vi "AMLUTwaveselHD2.vi"(0 "AM Freq Hz":dbl=1000.0, 5 "Peak Power":dbl=20.0, 7 "Min Power":dbl=10.0, 9 "Wave Shape":u8(ring) items=["Sine", "Ramp", "Triangle"], 12 "Linear in?":u8(ring) items=["Linear in dB", "Linear in Volts"]) -> (4 "Waveform":dbl[](graph), 8 "Actual Freq":dbl=1000.0, 13 "LUTsize":u8=32, 15 "powerout":string)   [LabVIEW 2012]
panel:
  out "stdam":u16
  # "dBm"
  # "dBm"
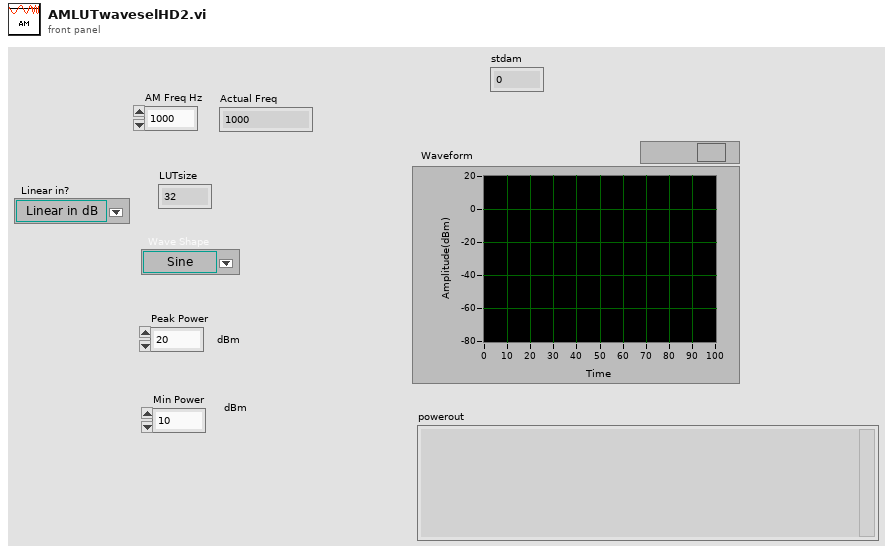
[diagram p1: front panel]
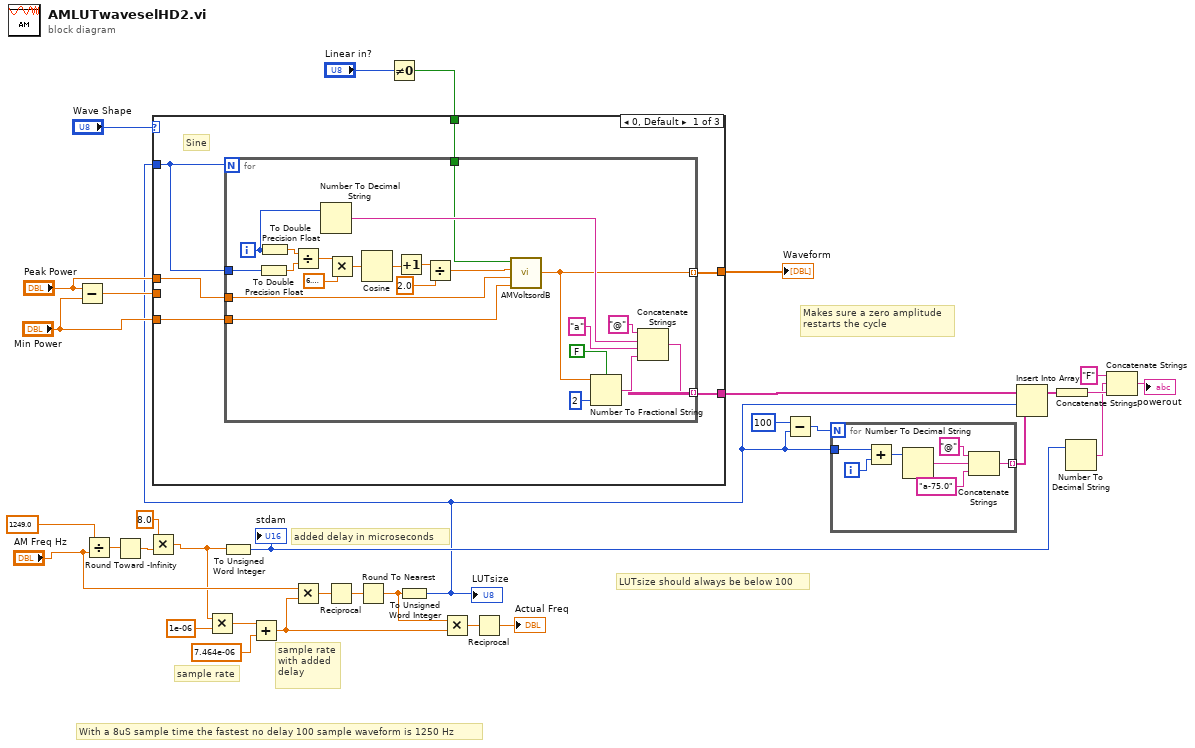
[diagram p0: block diagram]
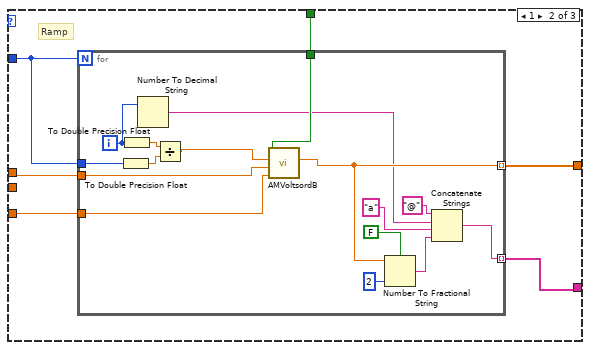
[diagram p2: hidden frame]
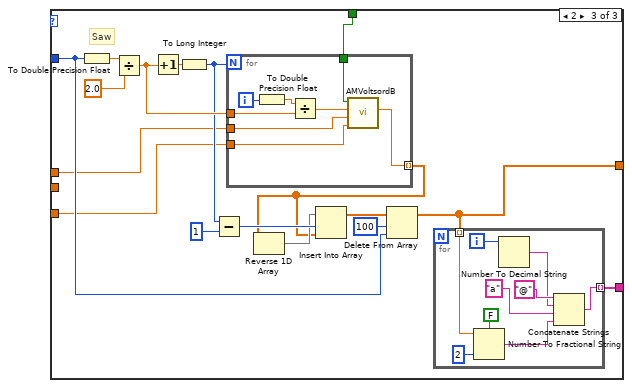
[diagram p3: hidden frame]
diagram:
  # "With a 8uS sample time the fastest no delay 100 sample waveform is 1250 Hz"
  # "LUTsize should always be below 100"
  # "added delay in microseconds"
  # "sample rate\nwith added\ndelay"
  # "sample rate"
  # "Makes sure a zero amplitude\nrestarts the cycle"
  n1 = Subtract(x="Peak Power", y="Min Power") -> (x-y=w32:dbl)
  n2 = Divide(x=1249.0, y="AM Freq Hz") -> (x/y=w11:dbl)
  n3 = Round Toward -Infinity(1:w11) -> (0:w10:dbl)
  n4 = Multiply(x=8.0, y=w10) -> (x*y=w9:dbl)
  n5 = Multiply(x=w9, y=1e-06) -> (x*y=w21:dbl)
  n6 = To Unsigned Word Integer(number=w9) -> (unsigned 16bit integer=w24:u16)
  "stdam" <- w24
  n7 = Add(x=w21, y=7.464e-06 ("x")) -> (x+y=w13:dbl)
  n8 = Multiply(x="AM Freq Hz", y=w13) -> (x*y=w19:dbl)
  n9 = Reciprocal(x=w19) -> (1/x=w18:dbl)
  n10 = Round To Nearest(number=w18) -> (nearest integer value=w14:dbl)
  n11 = Not Equal To 0?(x="Linear in?") -> (x != 0?=w5:bool)
  n12 = To Unsigned Word Integer(number=w14) -> (unsigned 16bit integer=w2:u16)
  "LUTsize" <- w2
  n13 = case shown="0, Default" "Wave Shape" {
    tunnel: [w38 w67 w89] -> w7
    tunnel: w2 -> [w39 w66 w92]
    tunnel: "Min Power" -> [w37 w65 w90]
    tunnel: [w36 w64 w88] -> w30
    tunnel: w32 -> [_ _ _]
    tunnel: w5 -> [w35 w63 w86]
    tunnel: "Peak Power" -> [w34 w62 w87]
    frame 0, Default {
      # "Sine"
      n14 = for {
        N: w39 -> [_]
        tunnel: [w42] -> w38 mode=indexing
        tunnel: w39 -> [w56]
        tunnel: w37 -> [w49]
        tunnel: [w52] -> w36 mode=indexing
        tunnel: w35 -> [w51]
        tunnel: w34 -> [w50]
        i -> [w55]
        n15 = To Double Precision Float(number=w56) -> (double precision float=w57:dbl)
        n16 = To Double Precision Float(number=w55) -> (double precision float=w58:dbl)
        n17 = Divide(x=w58, y=w57) -> (x/y=w61:dbl)
        n18 = Number To Decimal String(number=w55) -> (decimal integer string=w54:string)  [unwired: 1 in]
        n19 = Multiply(x=w61, y=6.283185307179586) -> (x*y=w59:dbl)
        n20 = Cosine(x=w59) -> (cos(x)=w48:dbl)
        n21 = Increment(x=w48) -> (x+1=w47:dbl)
        n22 = Divide(x=w47, y=2.0) -> (x/y=w45:dbl)
        n23 = call "AMVoltsordB.vi"("Min Power"=w49, "Peak Power"=w50, "Signal In"=w45, "Linear?"=w51) -> ("Out"=w42:dbl)  [unwired: 7 in]
        n24 = Number To Fractional String(use system decimal point (T)=FALSE, number=w42, precision (6)=i16 2) -> (F-format string=w43:string)  [unwired: 1 in]
        n25 = Concatenate Strings("@" ("string"), w54, "a" ("string"), w43) -> (w52:string)
      }
    }
    frame 1 {
      # "Ramp"
      n26 = for {
        N: w66 -> [_]
        tunnel: [w70] -> w67 mode=indexing
        tunnel: w66 -> [w81]
        tunnel: w62 -> [w78]
        tunnel: w65 -> [w79]
        tunnel: [w68] -> w64 mode=indexing
        tunnel: w63 -> [w77]
        i -> [w80]
        n27 = To Double Precision Float(number=w81) -> (double precision float=w82:dbl)
        n28 = To Double Precision Float(number=w80) -> (double precision float=w83:dbl)
        n29 = Number To Decimal String(number=w80) -> (decimal integer string=w69:string)  [unwired: 1 in]
        n30 = Divide(x=w83, y=w82) -> (x/y=w76:dbl)
        n31 = call "AMVoltsordB.vi"("Min Power"=w79, "Peak Power"=w78, "Signal In"=w76, "Linear?"=w77) -> ("Out"=w70:dbl)  [unwired: 7 in]
        n32 = Number To Fractional String(use system decimal point (T)=FALSE, number=w70, precision (6)=i16 2) -> (F-format string=w73:string)  [unwired: 1 in]
        n33 = Concatenate Strings("@" ("string"), w69, "a" ("string"), w73) -> (w68:string)
      }
    }
    frame 2 {
      # "Saw"
      n34 = To Double Precision Float(number=w92) -> (double precision float=w100:dbl)
      n35 = Divide(x=w100, y=2.0) -> (x/y=w97:dbl)
      n36 = Increment(x=w97) -> (x+1=w98:dbl)
      n37 = To Long Integer(number=w98) -> (32bit integer=w96:i32)
      n38 = Subtract(x=w96, y=1) -> (x-y=w95:i32)
      n39 = for {
        N: w96 -> [_]
        tunnel: [w110] -> w84 mode=indexing
        tunnel: w97 -> [w115]
        tunnel: w87 -> [w112]
        tunnel: w90 -> [w113]
        tunnel: w86 -> [w111]
        i -> [w116]
        n40 = To Double Precision Float(number=w116) -> (double precision float=w117:dbl)
        n41 = Divide(x=w117, y=w115) -> (x/y=w114:dbl)
        n42 = call "AMVoltsordB.vi"("Min Power"=w113, "Peak Power"=w112, "Signal In"=w114, "Linear?"=w111) -> ("Out"=w110:dbl)  [unwired: 7 in]
      }
      n43 = Reverse 1D Array(array=w84) -> (reversed array=w85:dbl[])
      n44 = Insert Into Array(array=w85, index=w95, new element=w84) -> (w93:dbl[])
      n45 = Delete From Array(array=w93, length=100, index=w92) -> (array with subset deleted=w89:dbl[])  [unwired: 1 out]
      n46 = for {
        tunnel: w89 -> [w102] mode=indexing
        tunnel: [w107] -> w88 mode=indexing
        i -> [w109]
        n47 = Number To Fractional String(use system decimal point (T)=FALSE, number=w102, precision (6)=i16 2) -> (F-format string=w101:string)  [unwired: 1 in]
        n48 = Number To Decimal String(number=w109) -> (decimal integer string=w106:string)  [unwired: 1 in]
        n49 = Concatenate Strings("@" ("string"), w106, "a" ("string"), w101) -> (w107:string)
      }
    }
  }
  "Waveform" <- w7
  n50 = Multiply(x=w14, y=w13) -> (x*y=w17:dbl)
  n51 = Reciprocal(x=w17) -> (1/x=→"Actual Freq":dbl)
  n52 = Subtract(x=u8 100 ("y"), y=w2) -> (x-y=w1:u16)
  n53 = for {
    N: w1 -> [_]
    tunnel: [w119] -> w4 mode=indexing
    tunnel: w2 -> [w118]
    i -> [w124]
    n54 = Add(x=w118, y=w124) -> (x+y=w120:i32)
    n55 = Number To Decimal String(number=w120) -> (decimal integer string=w122:string)  [unwired: 1 in]
    n56 = Concatenate Strings("@" ("string"), w122, "a-75.0" ("new element/subarray")) -> (w119:string)
  }
  n57 = Insert Into Array(array=w30, index=w2, new element=w4) -> (w29:string[])
  n58 = Concatenate Strings(w29) -> (w26:string)
  n59 = Number To Decimal String(number=w24) -> (decimal integer string=w25:string)  [unwired: 1 in]
  n60 = Concatenate Strings("F" ("string"), w25, w26) -> (→"powerout":string)
